vi "Get TimeStamp Formatted.vi"(8 "error in (no error)":errorcluster, 11 "Child_1 in":refnum<class "GUI_Class.lvclass">) -> (0 "error out":errorcluster, 1 "TimeStamp Formatted":string, 3 "Child_1 out":refnum<class "GUI_Class.lvclass">)   [LabVIEW 2023, in "GUI_Actor.lvlib" / "GUI_Class.lvclass"]
uses:
  GUI_Class.lvclass
  Abstraction_Interface_Class/Abstraction_Interface_Class.lvclass
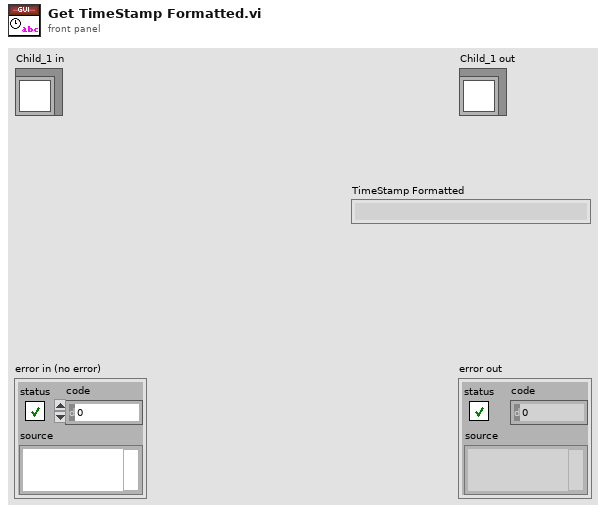
[diagram p1: front panel]
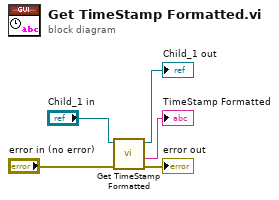
[diagram p0: block diagram]
diagram:
  n1 = call-parent "Get TimeStamp Formatted.vi"("error in (no error)"="error in (no error)", "Interface_Class in"="Child_1 in") -> ("error out"=→"error out":errorcluster, "TimeStamp Formatted"=→"TimeStamp Formatted":string, "Interface_Class out"=→"Child_1 out":refnum<class "GUI_Class.lvclass">)  [unwired: 7 in]
